vi "DAC Configure.vi"(8 "error in":errorcluster, 11 "DAC FTCU in":refnum<class "DAC FTCU.lvclass">) -> (0 "error out":errorcluster, 3 "DAC FTCU out":refnum<class "DAC FTCU.lvclass">)   [LabVIEW 2019, in "DAC.lvlib" / "DAC FTCU.lvclass"]
uses:
  DAC FTCU.lvclass
  C:/Users/wg/Documents/LV_Projects/test-stand/App/DAC/DAC.lvclass
  DAC.lvclass/DAC.ctl
  <vilib>/NI/Modbus Library/API/Master/Modbus Master.lvclass
  DAC FTCU.lvclass/DAC FTCU.ctl
  <vilib>/NI/Modbus Library/API/Wrapper/Create Serial Master.vi
  <vilib>/Utility/error.llb/Error Cluster From Error Code.vi
  <vilib>/ErrorRing/Error Ring.xnode
  DAC.lvclass
  <vilib>/NI/Modbus Library/API/Wrapper/API Main.lvlib
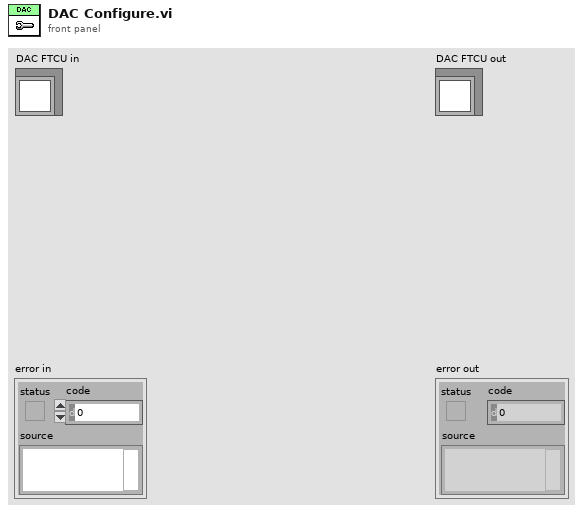
[diagram p1: front panel]
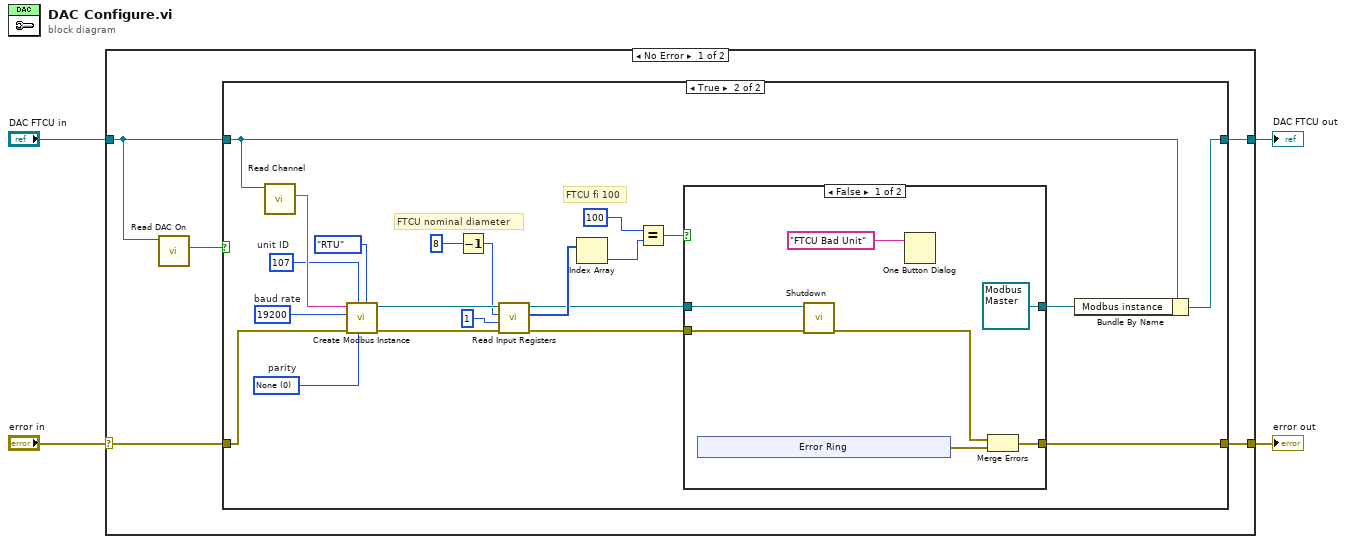
[diagram p0: block diagram]
diagram:
  n1 = case shown="No Error" "error in" {
    selector: "error in" -> [w6 w47]
    tunnel: [w5 w47] -> w4
    tunnel: [w7 w46] -> w3
    tunnel: "DAC FTCU in" -> [w9 w46]
    frame No Error {
      n2 = call "Read DAC On.vi"("DAC in"=w9) -> ("DAC On"=w8:bool)  [unwired: 8 in, 2 out]
      n3 = case shown="True" w8 {
        tunnel: w9 -> [w11 w31]
        tunnel: [w11 w32] -> w7
        tunnel: w6 -> [w10 w27]
        tunnel: [w10 w13] -> w5
        frame False {
        }
        frame True {
          w26 = u8 107  # unit ID
          w28 = u16 0 items=["None", "Odd", "Even", "Mark", "Space"]  # parity
          w29 = u32 19200  # baud rate
          # "FTCU fi 100"
          # "FTCU nominal diameter"
          n4 = call "Read Channel.vi"("DAC in"=w31) -> ("Channel"=w30:string)  [unwired: 8 in, 2 out]
          n5 = call-poly <vilib>:"Create Modbus Instance.vi"("serial type"=enum16{"RTU", "ASCII"}."RTU", "parity (even)"=w28, "unit ID"=w26, "error in"=w27, "baud rate"=w29, "VISA resource name"=w30) -> ("error out"=w20:errorcluster, "serial master instance"=w24:refnum<class "Modbus Master.lvclass">)  [unwired: 4 in]
          n6 = Decrement(x=u16 8 ("starting address")) -> (x-1=w22:u16)
          n7 = call-dynamic "Read Input Registers.vi"("error in"=w20, "number of inputs"=u16 1, "starting address"=w22, "Modbus master in"=w24) -> ("error out"=w12:errorcluster, "register values"=w18:u16[], "Modbus master out"=w15:refnum<class "Modbus Master.lvclass">)  [unwired: 5 in]
          n8 = Index Array(array=w18) -> (element=w17:u16)  [unwired: 1 in]
          n9 = Equal?(x=u16 100, y=w17) -> (x = y?=w16:bool)
          n10 = case shown="False" w16 {
            tunnel: w15 -> [w38 w45]
            tunnel: [refnum<class "Modbus Master.lvclass"> refnum ("Modbus master out") w45] -> w14
            tunnel: [w36 w44] -> w13
            tunnel: w12 -> [w37 w44]
            frame False {
              n11 = xnode "Error Ring"() -> ("error out"=w34:errorcluster)
              n12 = call-dynamic "Shutdown.vi"("error in"=w37, "Modbus master in"=w38) -> ("error out"=w35:errorcluster)  [unwired: 9 in]
              n13 = One Button Dialog(message="FTCU Bad Unit" ("format string")) -> ()  [unwired: 1 in, 1 out]
              n14 = Merge Errors(w35, w34) -> (w36:errorcluster)
            }
            frame True {
            }
          }
          n15 = Bundle By Name(cluster=w31, "Modbus instance"=w14) -> (w32:refnum<class "DAC FTCU.lvclass">)
        }
      }
    }
    frame Error {
    }
  }
  "error out" <- w4
  "DAC FTCU out" <- w3
